vi "Interpret Data - Byte.vi"(8 "error in (no error)":errorcluster, 9 "Byte order":T2, 10 "Action":T1, 11 "Data":u8 format="%02x") -> (0 "error out":errorcluster, 3 "Digital data bits":u8[](array[numeric]))   [LabVIEW 2009, in "IDW.lvlib"]
doc: "Changes a byte of binary data (bit states '1', '0') into digital waveform data, based on the desired action. \n\nThis is a polymorphic instance of the <b>Interpret Data</b> VI. For a <b>Transmit (Tx)</b> action, bits [1,0] are changed into [Z,0]. For a <b>Receive (Rx)</b> action, bits [1,0] are changed into [H,L].\n\nEach bit of the byte is added in the <b>Byte order</b> order, either MSB-first or LSB-first."
uses:
  IDW.lvlib
  _Typedefs/Byte order.ctl
  _Typedefs/Bus operation.ctl
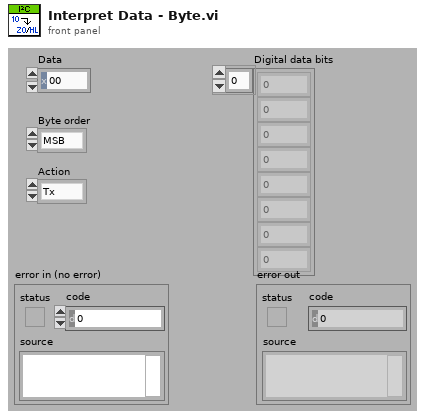
[diagram p1: front panel]
types:
  T1 = typedef "IDW.lvlib/Bus operation.ctl" = enum16{"Tx", "Rx"}
  T2 = typedef "IDW.lvlib/Byte order.ctl" = enum16{"MSB", "LSB"}
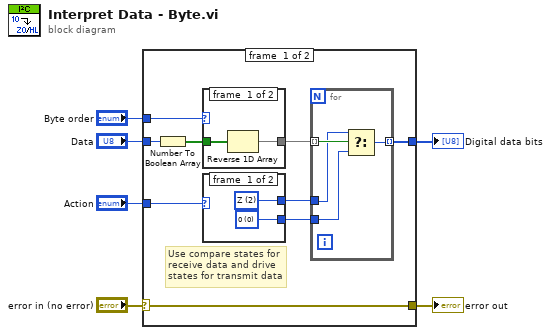
[diagram p0: block diagram]
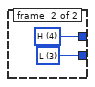
[diagram p2: hidden frame]
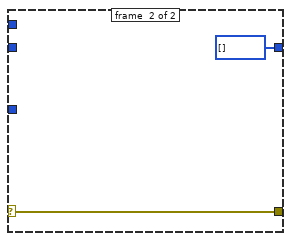
[diagram p4: hidden frame]
diagram:
  n1 = case shown="No Error" "error in (no error)" {
    selector: "error in (no error)" -> [w7 w27]
    tunnel: "Data" -> [w15 _]
    tunnel: "Byte order" -> [w12 _]
    tunnel: [w11 u8[] []] -> w4
    tunnel: "Action" -> [w8 _]
    tunnel: [w7 w27] -> w1
    frame #0 {
      # "Use compare states for receive data and drive states for transmit data"
      n2 = Number To Boolean Array(number=w15) -> (Boolean array=w14:bool[])
      n3 = case shown="\"MSB\", Default" w12 {
        tunnel: w14 -> [w25 w26]
        tunnel: [w24 w26] -> w13
        frame #0 {
          n4 = Reverse 1D Array(array=w25) -> (reversed array=w24:bool[])
        }
        frame #1 {
        }
      }
      n5 = case shown="\"Rx\"" w8 {
        tunnel: [w17 w19] -> w9
        tunnel: [w16 w18] -> w10
        frame #0 {
          w17 = u8 2 items=["0", "1", "Z", "L", "H", "X", "T", "V"] ("digital values ring")
          w16 = u8 0 items=["0", "1", "Z", "L", "H", "X", "T", "V"] ("digital values ring")
        }
        frame #1 {
          w19 = u8 4 items=["0", "1", "Z", "L", "H", "X", "T", "V"] ("digital values ring")
          w18 = u8 3 items=["0", "1", "Z", "L", "H", "X", "T", "V"] ("digital values ring")
        }
      }
      n6 = for {
        tunnel: w13 -> [w23] mode=indexing
        tunnel: [w22] -> w11 mode=indexing
        tunnel: w10 -> [w20]
        tunnel: w9 -> [w21]
        n7 = Select(t=w21, s=w23, f=w20) -> (s? t:f=w22:u8)
      }
    }
    frame #1 {
    }
  }
  "Digital data bits" <- w4
  "error out" <- w1
